vi "ui_initialize_connection.vi"(8 "error in (no error)":errorcluster caption="错误输入（无错误）", 11 "Controller Address":string caption="控制器地址") -> (0 "error out":errorcluster caption="错误输出", 2 "Connected?":bool caption="已连接？")   [LabVIEW 2015]
uses:
  message_queue/message_cluster.ctl
  type_definitions/variable_references.ctl
  globals/global_configuration_options.vi
  globals/global_ui_stream_and_variable_connections.vi
  message_queue/message_queue.lvlib
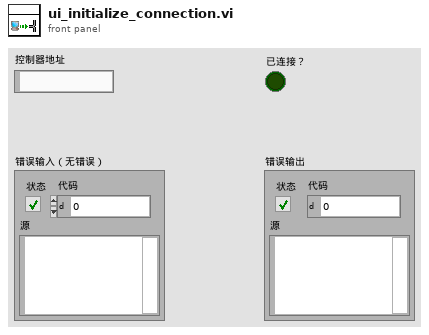
[diagram p1: front panel]
types:
  T1 = typedef "message_queue.lvlib/message_cluster.ctl" = cluster{"Message":string, "Message Data":variant}
  T2 = typedef "variable_references.ctl" = cluster{"CPU 1 Usage":refnum<k21>, "Free Memory":refnum<k21>, "Actual Loop Period":refnum<k21>, "CPU 2 Usage":refnum<k21>, "Drive Space":refnum<k21>, "Number of Data Files":refnum<k21>, "System Time":refnum<k21>}
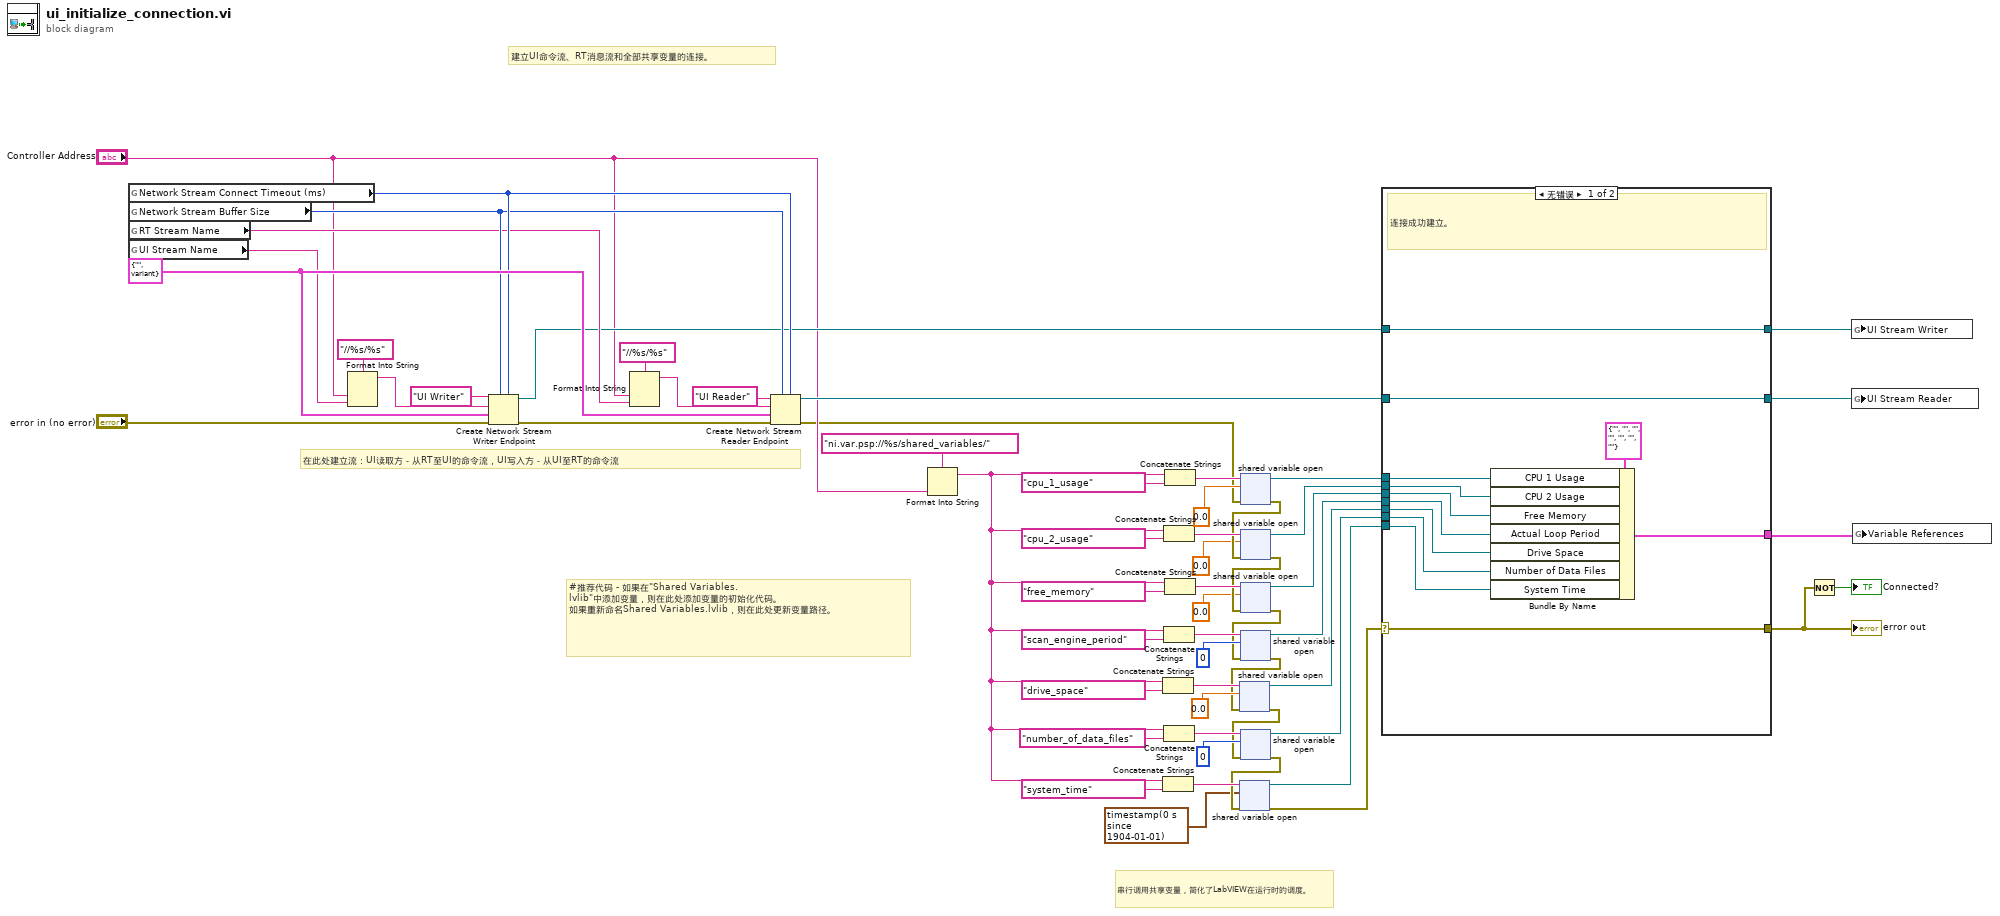
[diagram p0: block diagram]
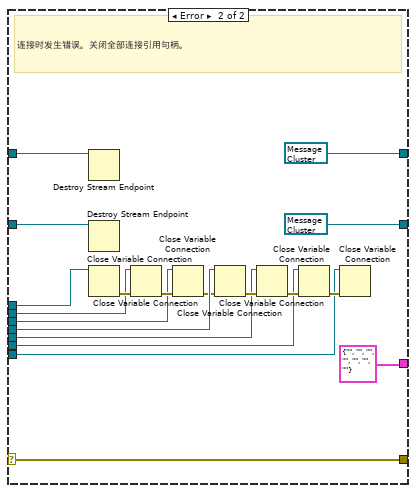
[diagram p2: hidden frame]
diagram:
  w53 = T1 {"Message"="", "Message Data"=variant} ("Message Cluster")
  # "建立UI命令流、RT消息流和全部共享变量的连接。"
  # "#推荐代码 - 如果在\"Shared Variables.lvlib\"中添加变量，则在此处添加变量的初始化代码。\n如果重新命名Shared Variables.lvlib，则在此处更新变量路径。"
  # "在此处建立流：UI读取方－从RT至UI的命令流，UI写入方－从UI至RT的命令流"
  # "串行调用共享变量，简化了LabVIEW在运行时的调度。"
  n1 = global read "global_configuration_options.vi" "Network Stream Connect Timeout (ms)"() -> (w51:i32)
  n2 = global read "global_configuration_options.vi" "Network Stream Buffer Size"() -> (w12:i32)
  n3 = global read "global_configuration_options.vi" "RT Stream Name"() -> (w9:string)
  n4 = global read "global_configuration_options.vi" "UI Stream Name"() -> (w10:string)
  n5 = Format Into String(format string="//%s/%s", "Controller Address", w10) -> (resulting string=w7:string)  [unwired: 2 in, 1 out]
  n6 = Create Network Stream Writer Endpoint(5:w51, 7:w12, 8:"error in (no error)", 9:w53, 10:w7, 11:"UI Writer" ("reader name")) -> (0:w52:errorcluster, 3:w6:refnum<k21>)  [unwired: 1 in]
  n7 = Format Into String(format string="//%s/%s", "Controller Address", w9) -> (resulting string=w8:string)  [unwired: 2 in, 1 out]
  n8 = Create Network Stream Reader Endpoint(5:w51, 7:w12, 8:w52, 9:w53, 10:w8, 11:"UI Reader" ("writer name")) -> (0:w2:errorcluster, 3:w34:refnum<k21>)  [unwired: 1 in]
  n9 = Format Into String(format string="ni.var.psp://%s/shared_variables/", "Controller Address") -> (resulting string=w5:string)  [unwired: 2 in, 1 out]
  n10 = Concatenate Strings(w5, "drive_space") -> (w27:string)
  n11 = Concatenate Strings(w5, "system_time") -> (w18:string)
  n12 = Concatenate Strings(w5, "cpu_2_usage") -> (w46:string)
  n13 = Concatenate Strings(w5, "scan_engine_period") -> (w42:string)
  n14 = Concatenate Strings(w5, "number_of_data_files") -> (w21:string)
  n15 = Concatenate Strings(w5, "cpu_1_usage") -> (w49:string)
  n16 = Concatenate Strings(w5, "free_memory") -> (w45:string)
  n17 = shared-variable-open(w49, w2, 0.0) -> (w38:refnum<k21>, w40:errorcluster)  [unwired: 1 in]
  n18 = shared-variable-open(w46, w40, 0.0) -> (w37:refnum<k21>, w39:errorcluster)  [unwired: 1 in]
  n19 = shared-variable-open(w45, w39, 0.0) -> (w36:refnum<k21>, w30:errorcluster)  [unwired: 1 in]
  n20 = shared-variable-open(w42, w30, u32 0) -> (w35:refnum<k21>, w26:errorcluster)  [unwired: 1 in]
  n21 = shared-variable-open(w27, w26, 0.0) -> (w25:refnum<k21>, w20:errorcluster)  [unwired: 1 in]
  n22 = shared-variable-open(w21, w20, u32 0) -> (w19:refnum<k21>, w17:errorcluster)  [unwired: 1 in]
  n23 = shared-variable-open(w18, w17, timestamp(0 s since 1904-01-01) ("time stamp")) -> (w15:refnum<k21>, w16:errorcluster)  [unwired: 1 in]
  n24 = case shown="无错误" w16 {
    selector: w16 -> [w60 w72]
    tunnel: w38 -> [w70 w86]
    tunnel: w37 -> [w69 w83]
    tunnel: w36 -> [w68 w84]
    tunnel: w35 -> [w67 w85]
    tunnel: w34 -> [w64 w89]
    tunnel: w6 -> [w65 w90]
    tunnel: [w66 T2 {"CPU 1 Usage"="", "Free Memory"="", "Actual Loop Period"="", "CPU 2 Usage"="", "Drive Space"="", "Number of Data Files"="", "System Time"=""} ("Variable References")] -> w33
    tunnel: [w65 refnum<k21> refnum] -> w32
    tunnel: [w64 refnum<k21> refnum] -> w31
    tunnel: w25 -> [w63 w79]
    tunnel: w19 -> [w62 w77]
    tunnel: w15 -> [w61 w75]
    tunnel: [w60 w72] -> w1
    frame No Error {
      # "连接成功建立。"
      n25 = Bundle By Name(cluster=T2 {"CPU 1 Usage"="", "Free Memory"="", "Actual Loop Period"="", "CPU 2 Usage"="", "Drive Space"="", "Number of Data Files"="", "System Time"=""} ("Variable References"), "CPU 1 Usage"=w70, "CPU 2 Usage"=w69, "Free Memory"=w68, "Actual Loop Period"=w67, "Drive Space"=w63, "Number of Data Files"=w62, "System Time"=w61) -> (w66:T2)
    }
    frame Error {
      # "连接时发生错误。关闭全部连接引用句柄。"
      n26 = Destroy Stream Endpoint(11:w90) -> ()  [unwired: 1 in, 1 out]
      n27 = Destroy Stream Endpoint(11:w89) -> ()  [unwired: 1 in, 1 out]
      n28 = Close Variable Connection(11:w86) -> (0:w87:errorcluster)  [unwired: 1 in]
      n29 = Close Variable Connection(8:w87, 11:w83) -> (0:w88:errorcluster)
      n30 = Close Variable Connection(8:w88, 11:w84) -> (0:w81:errorcluster)
      n31 = Close Variable Connection(8:w81, 11:w85) -> (0:w80:errorcluster)
      n32 = Close Variable Connection(8:w80, 11:w79) -> (0:w78:errorcluster)
      n33 = Close Variable Connection(8:w78, 11:w77) -> (0:w76:errorcluster)
      n34 = Close Variable Connection(8:w76, 11:w75) -> ()  [unwired: 1 out]
    }
  }
  "error out" <- w1
  n35 = Not(x=w1) -> (.not. x?=→"Connected?":bool)
  n36 = global write "global_ui_stream_and_variable_connections.vi" "UI Stream Writer"(w32) -> ()
  n37 = global write "global_ui_stream_and_variable_connections.vi" "UI Stream Reader"(w31) -> ()
  n38 = global write "global_ui_stream_and_variable_connections.vi" "Variable References"(w33) -> ()
